vi "Read Both Fans Fault and State.vi"(8 "error in (no error)":errorcluster, 11 "Dual Fan in":refnum<class "Dual Fan.lvclass">) -> (0 "error out":errorcluster, 1 "Fan B Fault":bool, 2 "Fan B State":bool, 3 "Fan A Fault":bool, 5 "Fan A State":bool)   [LabVIEW 2018, in "Dual Fan.lvlib" / "Dual Fan.lvclass"]
doc: "Child classes should override this method to read information about the two fans: fault and state (aka whether the fan is on or not)."
uses:
  Dual Fan.lvclass
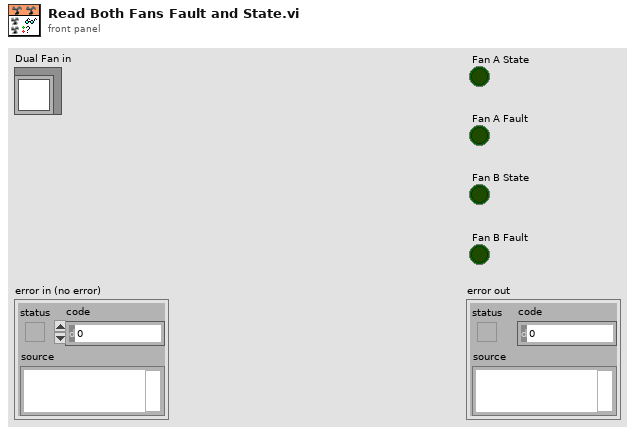
[diagram p1: front panel]
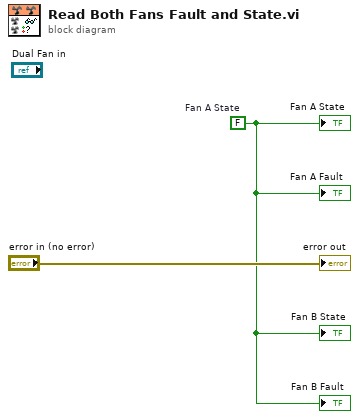
[diagram p0: block diagram]
diagram:
  w1 = FALSE  # Fan A State
  "Fan A Fault" <- w1
  "error out" <- "error in (no error)"
  "Fan B Fault" <- w1
  "Fan B State" <- w1
  "Fan A State" <- w1
